vi "ORS_linearize_Hilbert.vi"(7 "# zeros added":i32, 9 "Ch1 Michelson":dbl[](array[numeric]), 10 "Hilbert in":dbl[](array[numeric]), 11 "interpolation method":i32(ring)=1 caption="method" items=["nächste", "linear", "Spline", "Hermite (kubisch)", "Lagrange"]) -> (4 "error count":i32, 5 "Ch1 linearized":dbl[](array[numeric]) format="%_6g")   [LabVIEW 2021]
uses:
  <vilib>/Analysis/1siggen.llb/Ramp Pattern by Samples.vi
  <vilib>/gmath/NI_Gmath.lvlib
  <vilib>/Analysis/NI_AALBase.lvlib
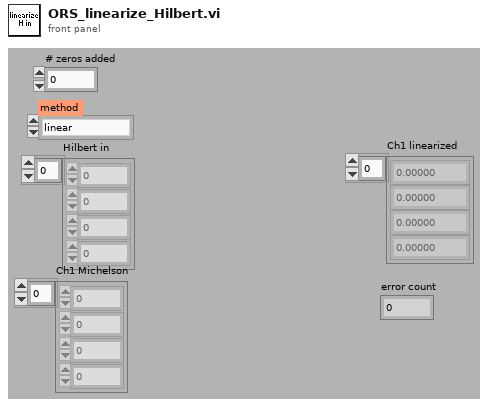
[diagram p1: front panel]
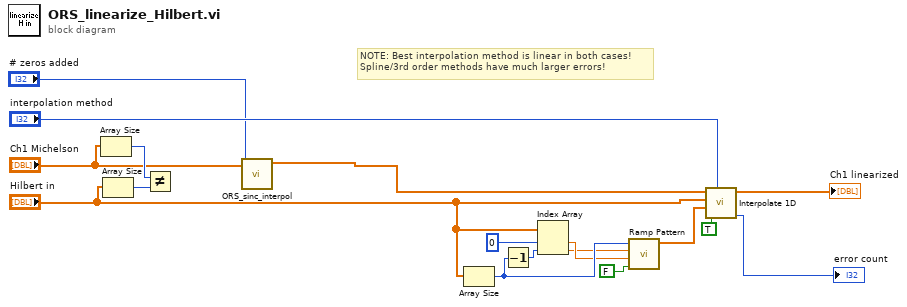
[diagram p0: block diagram]
diagram:
  # "NOTE: Best interpolation method is linear in both cases!\nSpline/3rd order methods have much larger errors!"
  n1 = Array Size(array="Ch1 Michelson") -> (size(s)=w13:i32)
  n2 = Array Size(array="Hilbert in") -> (size(s)=w12:i32)
  n3 = Not Equal?(x=w13, y=w12) -> ()  [unwired: 1 out]
  n4 = call "ORS_sinc_interpol.vi"("# zeros added"="# zeros added", "In"="Ch1 Michelson") -> ("Out"=w10:dbl[])  [unwired: 9 in]
  n5 = Array Size(array="Hilbert in") -> (size(s)=w5:i32)
  n6 = Decrement(x=w5) -> (x-1=w3:i32)
  n7 = Index Array(array="Hilbert in", index #1=0 ("index"), index #2=w3) -> (element #1=w2:dbl, element #2=w1:dbl)
  n8 = call-poly <vilib>:"Ramp Pattern.vi"("exclude end?"=FALSE, "start"=w2, "end"=w1, "samples"=w5) -> ("Ramp Pattern"=w8:dbl[])  [unwired: 6 in, 1 out]
  n9 = call <vilib>:"Interpolate 1D.vi"("method"="interpolation method", "X is monotonic"=TRUE, "xi"=w8, "X"="Hilbert in", "Y"=w10) -> ("error"=→"error count":i32, "yi"=→"Ch1 linearized":dbl[])  [unwired: 4 in, 1 out]
